vi "RSZVB Get Trace Transform Domain.vi"(8 "error in (no error)":errorcluster {"code" format="%.0x"}, 10 "Channel (Trace) (1)":i32=1, 11 "VISA session":refnum<visa-resource-name>) -> (0 "error out":errorcluster {"code" format="%.0x"}, 2 "Transform Domain":i32, 3 "dup VISA session":refnum<visa-resource-name>)   [LabVIEW 2011]
doc: "This VI queries the domain for active trace representation.\n\nRemote-control command(s):\nCALCulate<Ch/Tr>:TRANsform:TIME:STATe?"
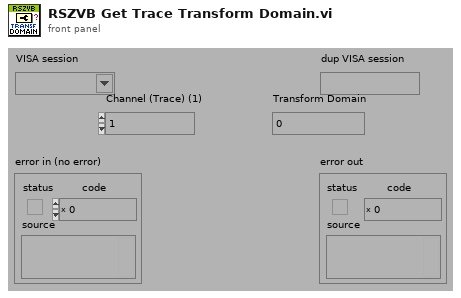
[diagram p1: front panel]
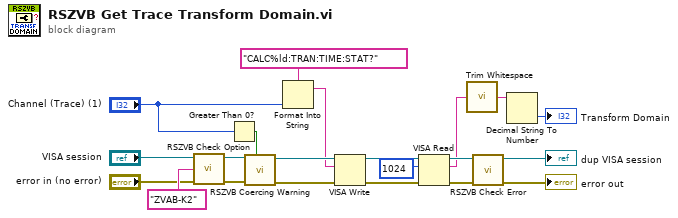
[diagram p0: block diagram]
diagram:
  n1 = call "RSZVB Check Option.vi"("error in (no error)"="error in (no error)", "Options"="ZVAB-K2", "VISA session"="VISA session") -> ("error out"=w7:errorcluster, "dup VISA session"=w6:refnum<visa-resource-name>)  [unwired: 7 in]
  n2 = Greater Than 0?(x="Channel (Trace) (1)") -> (x > 0?=w12:bool)
  n3 = call "RSZVB Coercing Warning.vi"("In Range?"=w12, "error in (no error)"=w7, "VISA session"=w6) -> ("error out"=w19:errorcluster, "dup VISA session"=w20:refnum<visa-resource-name>)  [unwired: 7 in]
  n4 = Format Into String(format string="CALC%ld:TRAN:TIME:STAT?", "Channel (Trace) (1)") -> (resulting string=w18:string)  [unwired: 2 in, 1 out]
  n5 = VISA Write(VISA resource name=w20, write buffer=w18, error in (no error)=w19) -> (VISA resource name out=w14:refnum<visa-resource-name>, error out=w13:errorcluster)  [unwired: 1 out]
  n6 = VISA Read(VISA resource name=w14, byte count=u32 1024 ("byte count (0)"), error in (no error)=w13) -> (VISA resource name out=w16:refnum<visa-resource-name>, read buffer=w3:string, error out=w15:errorcluster)  [unwired: 1 out]
  n7 = call <vilib>:"Trim Whitespace.vi"("string"=w3) -> ("trimmed string"=w2:string)  [unwired: 1 in]
  n8 = call "RSZVB Check Error.vi"("error in (no error)"=w15, "VISA session"=w16) -> ("error out"=→"error out":errorcluster, "dup VISA session"=→"dup VISA session":refnum<visa-resource-name>)  [unwired: 8 in]
  n9 = Decimal String To Number(string=w2) -> (number=→"Transform Domain":i32)  [unwired: 2 in, 1 out]
